vi "DoInit.vi"(8 "error in (no error)":errorcluster, 11 "Snake in":refnum<class "Snake.lvclass">) -> (0 "error out":errorcluster, 3 "Snake out":refnum<class "Snake.lvclass">)   [LabVIEW 2019, in "RT_Game.lvlib" / "Snake.lvclass"]
uses:
  Snake.lvclass
  Game/Coordinate.ctl
  Game/TileCodes.ctl
  Snake.lvclass/Snake.ctl
  Game/Game.lvclass
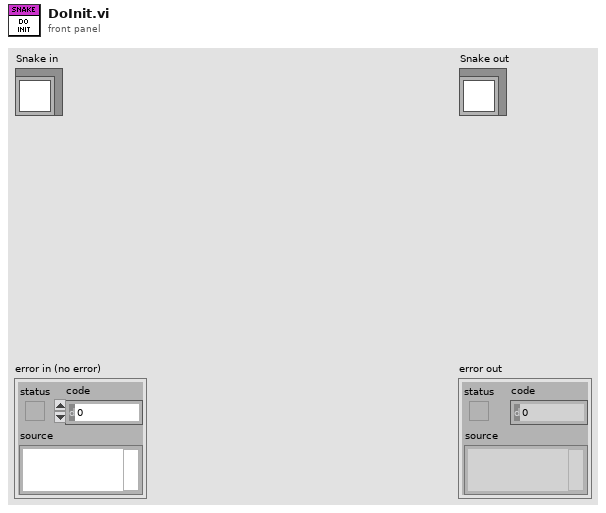
[diagram p1: front panel]
types:
  T1 = typedef "RT_Game.lvlib/Game.lvclass/Coordinate.ctl" = cluster{"x":i16, "y":i16}
  T2 = typedef "RT_Game.lvlib/Game.lvclass/TileCodes.ctl" = enum16{"line_vert", "line_hor", "line_rightup", "line_rightdown", "line_leftup", "line_leftdown", "bg1", "bg2", "bg3", "bg4", "bg5", "bg6", "bg7"}
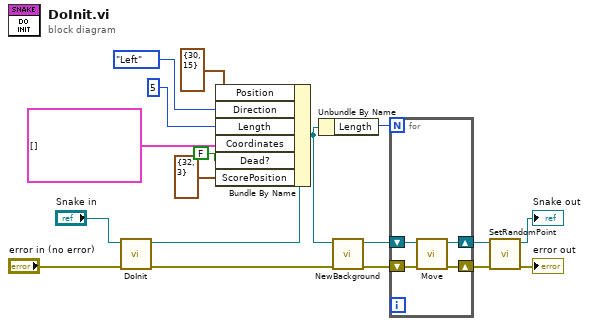
[diagram p0: block diagram]
diagram:
  n1 = call-parent "DoInit.vi"("error in (no error)"="error in (no error)", "Game in"="Snake in") -> ("error out"=w11:errorcluster, "Game out"=w18:refnum<class "Snake.lvclass">)  [unwired: 8 in]
  n2 = Bundle By Name(cluster=w18, "Position"=T1 {"x"=30, "y"=15}, "Direction"=enum16{"Up", "Down", "Left", "Right"}."Left", "Length"=i16 5, "Coordinates"=cluster{"Coordinate":T1, "TileCodes":T2}[] [], "Dead?"=FALSE, "ScorePosition"=T1 {"x"=32, "y"=3}) -> (w14:refnum<class "Snake.lvclass">)
  n3 = Unbundle By Name(w14) -> ("Length"=w13:i16)
  n4 = call "NewBackground.vi"("error in (no error)"=w11, "Snake in"=w14) -> ("error out"=w4:errorcluster, "Snake out"=w5:refnum<class "Snake.lvclass">)  [unwired: 8 in]
  n5 = for {
    N: w13 -> [_]
    shift-right: [w21] -> w8
    shift-left: w5 -> [w22]
    shift-right: [w19] -> w12
    shift-left: w4 -> [w20]
    n6 = call "Move.vi"("error in (no error)"=w20, "Snake in"=w22) -> ("error out"=w19:errorcluster, "Snake out"=w21:refnum<class "Snake.lvclass">)  [unwired: 8 in]
  }
  n7 = call "SetRandomPoint.vi"("error in (no error)"=w12, "Snake in"=w8) -> ("error out"=→"error out":errorcluster, "Snake out"=→"Snake out":refnum<class "Snake.lvclass">)  [unwired: 8 in]
